vi "op_num_v0.vi"() -> ()   [LabVIEW 2009]
panel:
  out "Afisare rezultat":dbl
  in  "Operand 2":dbl
  in  "Operand 1":dbl
  # "Aceasta aplicatie calculeaza produsul a doua numere\nintroduse de utilizator dupa care afiseaza rezultatul"
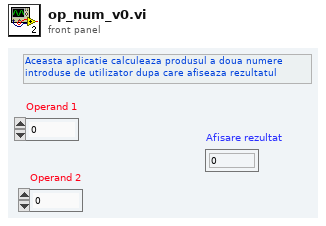
[diagram p1: front panel]
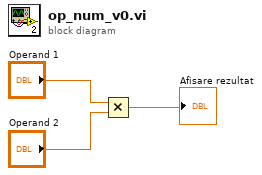
[diagram p0: block diagram]
diagram:
  n1 = Multiply(x="Operand 1", y="Operand 2") -> (x*y=→"Afisare rezultat":dbl)
